vi "nanocal -- nuclear schottky fit V8.vi"() -> ()   [LabVIEW 2021] (continued)
\"mm1\" -> 0.000097559485   ,  \"mm2\" -> 0.023589285914   ,  \"mm3\" -> 0.055607523989   ,  \"T\" -> 0.360000000000   ,  \"B\" -> 8.000000000000   ,  \"θ\" -> 0.000000000000   ,  \"Reoff\" -> -3448979.591836734680   ,  \"Imoff\" -> 0.000000000000   ,  \"στ1\" -> 0.000376669141   ,  \"στS\" -> 0.000017301947   ,  \"στN\" -> 0.000201176295   ,  \"τ11 \" -> 0.000000000000   ,  \"τ12\" -> 0.000000000000   ,  \"τ22\" -> 0.000000000000   ,  \"τN1\" -> 0.000000000000   ,  \"τN2\" -> 0.000000000000   ,  \"σηlogτ1 \" -> 0.000000000000   ,  \"σηlogτS\" -> 0.000000000000   ,  \"σηlogτN\" -> 0.000000000000   ,  \"σlogτ1\" -> 0.000000000000   ,  \"σlogτS\" -> 0.000000000000   ,  \"σlogτN\" -> 0.000000000000   ,  \"σητ1\" -> 0.000000000000   ,  \"σητS \" -> 0.000000000000   ,  \"σητN\" -> 0.000000000000    |>   , \r\"IDS0383_210910_RAW_cal__sam_\" ->   <|    \"ζ\" -> 0.038341835326   ,  \"τ1\" -> 0.050866858713   ,  \"τS\" -> 0.030652081909   ,  \"τN\" -> 0.004623805952   ,  \"τC\" -> 0.002823684758   ,  \"κ0\" -> 0.000000002289   ,  \"mm1\" -> 0.000096034779   ,  \"mm2\" -> 0.028459102290   ,  \"mm3\" -> 0.061763836547   ,  \"T\" -> 0.360000000000   ,  \"B\" -> 8.000000000000   ,  \"θ\" -> 0.000000000000   ,  \"Reoff\" -> 0.000000000000   ,  \"Imoff\" -> 0.000000000000   ,  \"στ1\" -> 0.000000000000   ,  \"στS\" -> 0.000000000000   ,  \"στN\" -> 0.000000000000   ,  \"τ11 \" -> 0.000000000000   ,  \"τ12\" -> 0.000000000000   ,  \"τ22\" -> 0.000000000000   ,  \"τN1\" -> 0.000000000000   ,  \"τN2\" -> 0.000000000000   ,  \"σηlogτ1 \" -> 0.000000000000   ,  \"σηlogτS\" -> 0.000000000000   ,  \"σηlogτN\" -> 0.000000000000   ,  \"σlogτ1\" -> 0.000000000000   ,  \"σlogτS\" -> 0.000000000000   ,  \"σlogτN\" -> 0.000000000000   ,  \"σητ1\" -> 0.000000000000   ,  \"σητS \" -> 0.000000000000   ,  \"σητN\" -> 0.000000000000    |>   , \r\"IDS0384_210910_RAW_cal__ref_\" ->   <|    \"ζ\" -> 0.048414028377   ,  \"τ1\" -> 0.045010611313   ,  \"τS\" -> 0.024057574241   ,  \"τN\" -> 0.002275401127   ,  \"τC\" -> 0.001753445489   ,  \"κ0\" -> 0.000000002628   ,  \"mm1\" -> 0.000075920940   ,  \"mm2\" -> 0.024140914114   ,  \"mm3\" -> 0.050155082533   ,  \"T\" -> 0.430000000000   ,  \"B\" -> 8.000000000000   ,  \"θ\" -> 0.000000000000   ,  \"Reoff\" -> -3244897.959183673380   ,  \"Imoff\" -> 0.000000000000   ,  \"στ1\" -> 0.000665063032   ,  \"στS\" -> 0.000021368158   ,  \"στN\" -> 0.000342578343   ,  \"τ11 \" -> 0.000000000000   ,  \"τ12\" -> 0.000000000000   ,  \"τ22\" -> 0.000000000000   ,  \"τN1\" -> 0.000000000000   ,  \"τN2\" -> 0.000000000000   ,  \"σηlogτ1 \" -> 0.000000000000   ,  \"σηlogτS\" -> 0.000000000000   ,  \"σηlogτN\" -> 0.000000000000   ,  \"σlogτ1\" -> 0.000000000000   ,  \"σlogτS\" -> 0.000000000000   ,  \"σlogτN\" -> 0.000000000000   ,  \"σητ1\" -> 0.000000000000   ,  \"σητS \" -> 0.000000000000   ,  \"σητN\" -> 0.000000000000    |>   , \r\"IDS0384_210910_RAW_cal__sam_\" ->   <|    \"ζ\" -> 0.029950572027   ,  \"τ1\" -> 0.044923259835   ,  \"τS\" -> 0.030416367718   ,  \"τN\" -> 0.002541256331   ,  \"τC\" -> 0.003331031560   ,  \"κ0\" -> 0.000000002858   ,  \"mm1\" -> 0.000087776347   ,  \"mm2\" -> 0.029544080465   ,  \"mm3\" -> 0.052567158325   ,  \"T\" -> 0.430000000000   ,  \"B\" -> 8.000000000000   ,  \"θ\" -> 0.000000000000   ,  \"Reoff\" -> 0.000000000000   ,  \"Imoff\" -> 0.000000000000   ,  \"στ1\" -> 0.000000000000   ,  \"στS\" -> 0.000000000000   ,  \"στN\" -> 0.000000000000   ,  \"τ11 \" -> 0.000000000000   ,  \"τ12\" -> 0.000000000000   ,  \"τ22\" -> 0.000000000000   ,  \"τN1\" -> 0.000000000000   ,  \"τN2\" -> 0.000000000000   ,  \"σηlogτ1 \" -> 0.000000000000   ,  \"σηlogτS\" -> 0.000000000000   ,  \"σηlogτN\" -> 0.000000000000   ,  \"σlogτ1\" -> 0.000000000000   ,  \"σlogτS\" -> 0.000000000000   ,  \"σlogτN\" -> 0.000000000000   ,  \"σητ1\" -> 0.000000000000   ,  \"σητS \" -> 0.000000000000   ,  \"σητN\" -> 0.000000000000    |>   , \r\"IDS0385_210910_RAW_cal__ref_\" ->   <|    \"ζ\" -> 0.037803233744   ,  \"τ1\" -> 0.038048590559   ,  \"τS\" -> 0.025073667725   ,  \"τN\" -> 0.001214857209   ,  \"τC\" -> 0.002021423784   ,  \"κ0\" -> 0.000000003274   ,  \"mm1\" -> 0.000068491984   ,  \"mm2\" -> 0.025433188254   ,  \"mm3\" -> 0.041850650292   ,  \"T\" -> 0.530000000000   ,  \"B\" -> 8.000000000000   ,  \"θ\" -> 0.000000000000   ,  \"Reoff\" -> -1979591.836734693500   ,  \"Imoff\" -> 0.000000000000   ,  \"στ1\" -> 0.001496353936   ,  \"στS\" -> 0.000028774209   ,  \"στN\" -> 0.000698641170   ,  \"τ11 \" -> 0.000000000000   ,  \"τ12\" -> 0.000000000000   ,  \"τ22\" -> 0.000000000000   ,  \"τN1\" -> 0.000000000000   ,  \"τN2\" -> 0.000000000000   ,  \"σηlogτ1 \" -> 0.000000000000   ,  \"σηlogτS\" -> 0.000000000000   ,  \"σηlogτN\" -> 0.000000000000   ,  \"σlogτ1\" -> 0.000000000000   ,  \"σlogτS\" -> 0.000000000000   ,  \"σlogτN\" -> 0.000000000000   ,  \"σητ1\" -> 0.000000000000   ,  \"σητS \" -> 0.000000000000   ,  \"σητN\" -> 0.000000000000    |>   , \r\"IDS0385_210910_RAW_cal__sam_\" ->   <|    \"ζ\" -> 0.024600756648   ,  \"τ1\" -> 0.043958236582   ,  \"τS\" -> 0.031312750224   ,  \"τN\" -> 0.001348105931   ,  \"τC\" -> 0.003635120795   ,  \"κ0\" -> 0.000000003548   ,  \"mm1\" -> 0.000078569164   ,  \"mm2\" -> 0.031960914170   ,  \"mm3\" -> 0.049018211972   ,  \"T\" -> 0.530000000000   ,  \"B\" -> 8.000000000000   ,  \"θ\" -> 0.000000000000   ,  \"Reoff\" -> 0.000000000000   ,  \"Imoff\" -> 0.000000000000   ,  \"στ1\" -> 0.000000000000   ,  \"στS\" -> 0.000000000000   ,  \"στN\" -> 0.000000000000   ,  \"τ11 \" -> 0.000000000000   ,  \"τ12\" -> 0.000000000000   ,  \"τ22\" -> 0.000000000000   ,  \"τN1\" -> 0.000000000000   ,  \"τN2\" -> 0.000000000000   ,  \"σηlogτ1 \" -> 0.000000000000   ,  \"σηlogτS\" -> 0.000000000000   ,  \"σηlogτN\" -> 0.000000000000   ,  \"σlogτ1\" -> 0.000000000000   ,  \"σlogτS\" -> 0.000000000000   ,  \"σlogτN\" -> 0.000000000000   ,  \"σητ1\" -> 0.000000000000   ,  \"σητS \" -> 0.000000000000   ,  \"σητN\" -> 0.000000000000    |>   , \r\"IDS0386_210910_RAW_cal__ref_\" ->   <|    \"ζ\" -> 0.027746649612   ,  \"τ1\" -> 0.033747008640   ,  \"τS\" -> 0.026895844648   ,  \"τN\" -> 0.000802809162   ,  \"τC\" -> 0.002381968002   ,  \"κ0\" -> 0.000000003893   ,  \"mm1\" -> 0.000059322452   ,  \"mm2\" -> 0.026788808143   ,  \"mm3\" -> 0.037748044699   ,  \"T\" -> 0.630000000000   ,  \"B\" -> 8.000000000000   ,  \"θ\" -> 0.000000000000   ,  \"Reoff\" -> -918367.346938774919   ,  \"Imoff\" -> 0.000000000000   ,  \"στ1\" -> 0.002776813512   ,  \"στS\" -> 0.000037245612   ,  \"στN\" -> 0.001225903353   ,  \"τ11 \" -> 0.000000000000   ,  \"τ12\" -> 0.000000000000   ,  \"τ22\" -> 0.000000000000   ,  \"τN1\" -> 0.000000000000   ,  \"τN2\" -> 0.000000000000   ,  \"σηlogτ1 \" -> 0.000000000000   ,  \"σηlogτS\" -> 0.000000000000   ,  \"σηlogτN\" -> 0.000000000000   ,  \"σlogτ1\" -> 0.000000000000   ,  \"σlogτS\" -> 0.000000000000   ,  \"σlogτN\" -> 0.000000000000   ,  \"σητ1\" -> 0.000000000000   ,  \"σητS \" -> 0.000000000000   ,  \"σητN\" -> 0.000000000000    |>   , \r\"IDS0386_210910_RAW_cal__sam_\" ->   <|    \"ζ\" -> 0.019494767421   ,  \"τ1\" -> 0.040349410363   ,  \"τS\" -> 0.033202805363   ,  \"τN\" -> 0.000770756985   ,  \"τC\" -> 0.004303152006   ,  \"κ0\" -> 0.000000004241   ,  \"mm1\" -> 0.000073144130   ,  \"mm2\" -> 0.033928832906   ,  \"mm3\" -> 0.045286454378   ,  \"T\" -> 0.630000000000   ,  \"B\" -> 8.000000000000   ,  \"θ\" -> 0.000000000000   ,  \"Reoff\" -> 0.000000000000   ,  \"Imoff\" -> 0.000000000000   ,  \"στ1\" -> 0.000000000000   ,  \"στS\" -> 0.000000000000   ,  \"στN\" -> 0.000000000000   ,  \"τ11 \" -> 0.000000000000   ,  \"τ12\" -> 0.000000000000   ,  \"τ22\" -> 0.000000000000   ,  \"τN1\" -> 0.000000000000   ,  \"τN2\" -> 0.000000000000   ,  \"σηlogτ1 \" -> 0.000000000000   ,  \"σηlogτS\" -> 0.000000000000   ,  \"σηlogτN\" -> 0.000000000000   ,  \"σlogτ1\" -> 0.000000000000   ,  \"σlogτS\" -> 0.000000000000   ,  \"σlogτN\" -> 0.000000000000   ,  \"σητ1\" -> 0.000000000000   ,  \"σητS \" -> 0.000000000000   ,  \"σητN\" -> 0.000000000000    |>   , \r\"IDS0387_210910_RAW_cal__ref_\" ->   <|    \"ζ\" -> 0.019313601846   ,  \"τ1\" -> 0.030127940029   ,  \"τS\" -> 0.030834079671   ,  \"τN\" -> 0.000314036282   ,  \"τC\" -> 0.003752610189   ,  \"κ0\" -> 0.000000005418   ,  \"mm1\" -> 0.000063634095   ,  \"mm2\" -> 0.028697652257   ,  \"mm3\" -> 0.036868962129   ,  \"T\" -> 0.830000000000   ,  \"B\" -> 8.000000000000   ,  \"θ\" -> 0.000000000000   ,  \"Reoff\" -> -265306.122448978945   ,  \"Imoff\" -> 0.000000000000   ,  \"στ1\" -> 0.011424377975   ,  \"στS\" -> 0.000061541841   ,  \"στN\" -> 0.005052534408   ,  \"τ11 \" -> 0.000000000000   ,  \"τ12\" -> 0.000000000000   ,  \"τ22\" -> 0.000000000000   ,  \"τN1\" -> 0.000000000000   ,  \"τN2\" -> 0.000000000000   ,  \"σηlogτ1 \" -> 0.000000000000   ,  \"σηlogτS\" -> 0.000000000000   ,  \"σηlogτN\" -> 0.000000000000   ,  \"σlogτ1\" -> 0.000000000000   ,  \"σlogτS\" -> 0.000000000000   ,  \"σlogτN\" -> 0.000000000000   ,  \"σητ1\" -> 0.000000000000   ,  \"σητS \" -> 0.000000000000   ,  \"σητN\" -> 0.000000000000    |>   , \r\"IDS0387_210910_RAW_cal__sam_\" ->   <|    \"ζ\" -> 0.013958531253   ,  \"τ1\" -> 0.040449551738   ,  \"τS\" -> 0.038075316972   ,  \"τN\" -> 0.000218997482   ,  \"τC\" -> 0.005348147372   ,  \"κ0\" -> 0.000000005866   ,  \"mm1\" -> 0.000064761782   ,  \"mm2\" -> 0.038768935960   ,  \"mm3\" -> 0.045792848207   ,  \"T\" -> 0.830000000000   ,  \"B\" -> 8.000000000000   ,  \"θ\" -> 0.000000000000   ,  \"Reoff\" -> 0.000000000000   ,  \"Imoff\" -> 0.000000000000   ,  \"στ1\" -> 0.000000000000   ,  \"στS\" -> 0.000000000000   ,  \"στN\" -> 0.000000000000   ,  \"τ11 \" -> 0.000000000000   ,  \"τ12\" -> 0.000000000000   ,  \"τ22\" -> 0.000000000000   ,  \"τN1\" -> 0.000000000000   ,  \"τN2\" -> 0.000000000000   ,  \"σηlogτ1 \" -> 0.000000000000   ,  \"σηlogτS\" -> 0.000000000000   ,  \"σηlogτN\" -> 0.000000000000   ,  \"σlogτ1\" -> 0.000000000000   ,  \"σlogτS\" -> 0.000000000000   ,  \"σlogτN\" -> 0.000000000000   ,  \"σητ1\" -> 0.000000000000   ,  \"σητS \" -> 0.000000000000   ,  \"σητN\" -> 0.000000000000    |>   , \r\"IDS0388_210910_RAW_cal__ref_\" ->   <|    \"ζ\" -> 0.016319215592   ,  \"τ1\" -> 0.028476907475   ,  \"τS\" -> 0.040634863110   ,  \"τN\" -> 0.000119778793   ,  \"τC\" -> 0.003363489331   ,  \"κ0\" -> 0.000000007540   ,  \"mm1\" -> 0.000049996694   ,  \"mm2\" -> 0.028266417043   ,  \"mm3\" -> 0.044943708759   ,  \"T\" -> 1.130000000000   ,  \"B\" -> 8.000000000000   ,  \"θ\" -> 0.000000000000   ,  \"Reoff\" -> -428571.428571428172   ,  \"Imoff\" -> 0.000000000000   ,  \"στ1\" -> 0.056097814520   ,  \"στS\" -> 0.000101338732   ,  \"στN\" -> 0.027741009439   ,  \"τ11 \" -> 0.000000000000   ,  \"τ12\" -> 0.000000000000   ,  \"τ22\" -> 0.000000000000   ,  \"τN1\" -> 0.000000000000   ,  \"τN2\" -> 0.000000000000   ,  \"σηlogτ1 \" -> 0.000000000000   ,  \"σηlogτS\" -> 0.000000000000   ,  \"σηlogτN\" -> 0.000000000000   ,  \"σlogτ1\" -> 0.000000000000   ,  \"σlogτS\" -> 0.000000000000   ,  \"σlogτN\" -> 0.000000000000   ,  \"σητ1\" -> 0.000000000000   ,  \"σητS \" -> 0.000000000000   ,  \"σητN\" -> 0.000000000000    |>   , \r\"IDS0388_210910_RAW_cal__sam_\" ->   <|    \"ζ\" -> 0.011551866824   ,  \"τ1\" -> 0.040411227639   ,  \"τS\" -> 0.048181354691   ,  \"τN\" -> 0.000103559724   ,  \"τC\" -> 0.006232382617   ,  \"κ0\" -> 0.000000008161   ,  \"mm1\" -> 0.000063176601   ,  \"mm2\" -> 0.040126882627   ,  \"mm3\" -> 0.055296246344   ,  \"T\" -> 1.130000000000   ,  \"B\" -> 8.000000000000   ,  \"θ\" -> 0.000000000000   ,  \"Reoff\" -> 0.000000000000   ,  \"Imoff\" -> 0.000000000000   ,  \"στ1\" -> 0.000000000000   ,  \"στS\" -> 0.000000000000   ,  \"στN\" -> 0.000000000000   ,  \"τ11 \" -> 0.000000000000   ,  \"τ12\" -> 0.000000000000   ,  \"τ22\" -> 0.000000000000   ,  \"τN1\" -> 0.000000000000   ,  \"τN2\" -> 0.000000000000   ,  \"σηlogτ1 \" -> 0.000000000000   ,  \"σηlogτS\" -> 0.000000000000   ,  \"σηlogτN\" -> 0.000000000000   ,  \"σlogτ1\" -> 0.000000000000   ,  \"σlogτS\" -> 0.000000000000   ,  \"σlogτN\" -> 0.000000000000   ,  \"σητ1\" -> 0.000000000000   ,  \"σητS \" -> 0.000000000000   ,  \"σητN\" -> 0.000000000000    |>   , \r\"IDS0389_210910_RAW_cal__ref_\" ->   <|    \"ζ\" -> 0.019598304636   ,  \"τ1\" -> 0.026919422871   ,  \"τS\" -> 0.016301457757   ,  \"τN\" -> 0.000045685674   ,  \"τC\" -> 0.003967911941   ,  \"κ0\" -> 0.000000010417   ,  \"mm1\" -> 0.000061755971   ,  \"mm2\" -> 0.020381971483   ,  \"mm3\" -> 0.027111127086   ,  \"T\" -> 1.520000000000   ,  \"B\" -> 8.000000000000   ,  \"θ\" -> 0.000000000000   ,  \"Reoff\" -> -551020.408163265324   ,  \"Imoff\" -> 0.000000000000   ,  \"στ1\" -> 0.092677427953   ,  \"στS\" -> 0.000105745650   ,  \"στN\" -> 0.043266676347   ,  \"τ11 \" -> 0.000000000000   ,  \"τ12\" -> 0.000000000000   ,  \"τ22\" -> 0.000000000000   ,  \"τN1\" -> 0.000000000000   ,  \"τN2\" -> 0.000000000000   ,  \"σηlogτ1 \" -> 0.000000000000   ,  \"σηlogτS\" -> 0.000000000000   ,  \"σηlogτN\" -> 0.000000000000   ,  \"σlogτ1\" -> 0.000000000000   ,  \"σlogτS\" -> 0.000000000000   ,  \"σlogτN\" -> 0.000000000000   ,  \"σητ1\" -> 0.000000000000   ,  \"σητS \" -> 0.000000000000   ,  \"σητN\" -> 0.000000000000    |>   , \r\"IDS0389_210910_RAW_cal__sam_\" ->   <|    \"ζ\" -> 0.011148198813   ,  \"τ1\" -> 0.038849151842   ,  \"τS\" -> 0.019213865355   ,  \"τN\" -> 0.000045035153   ,  \"τC\" -> 0.005536708133   ,  \"κ0\" -> 0.000000011229   ,  \"mm1\" -> 0.000047596165   ,  \"mm2\" -> 0.024836509281   ,  \"mm3\" -> 0.038975357089   ,  \"T\" -> 1.520000000000   ,  \"B\" -> 8.000000000000   ,  \"θ\" -> 0.000000000000   ,  \"Reoff\" -> 0.000000000000   ,  \"Imoff\" -> 0.000000000000   ,  \"στ1\" -> 0.000000000000   ,  \"στS\" -> 0.000000000000   ,  \"στN\" -> 0.000000000000   ,  \"τ11 \" -> 0.000000000000   ,  \"τ12\" -> 0.000000000000   ,  \"τ22\" -> 0.000000000000   ,  \"τN1\" -> 0.000000000000   ,  \"τN2\" -> 0.000000000000   ,  \"σηlogτ1 \" -> 0.000000000000   ,  \"σηlogτS\" -> 0.000000000000   ,  \"σηlogτN\" -> 0.000000000000   ,  \"σlogτ1\" -> 0.000000000000   ,  \"σlogτS\" -> 0.000000000000   ,  \"σlogτN\" -> 0.000000000000   ,  \"σητ1\" -> 0.000000000000   ,  \"σητS \" -> 0.000000000000   ,  \"σητN\" -> 0.000000000000    |>   , \r\"IDS0390_210910_RAW_cal__ref_\" ->   <|    \"ζ\" -> 0.016930911493   ,  \"τ1\" -> 0.024035041541   ,  \"τS\" -> 0.011182752166   ,  \"τN\" -> 0.000024854278   ,  \"τC\" -> 0.003445627696   ,  \"κ0\" -> 0.000000013051   ,  \"mm1\" -> 0.000044158259   ,  \"mm2\" -> 0.014733556006   ,  \"mm3\" -> 0.024100316408   ,  \"T\" -> 1.900000000000   ,  \"B\" -> 8.000000000000   ,  \"θ\" -> 0.000000000000   ,  \"Reoff\" -> -346938.775510204024   ,  \"Imoff\" -> 0.000000000000   ,  \"στ1\" -> 0.156695414704   ,  \"στS\" -> 0.000120966838   ,  \"στN\" -> 0.078791038522   ,  \"τ11 \" -> 0.000000000000   ,  \"τ12\" -> 0.000000000000   ,  \"τ22\" -> 0.000000000000   ,  \"τN1\" -> 0.000000000000   ,  \"τN2\" -> 0.000000000000   ,  \"σηlogτ1 \" -> 0.000000000000   ,  \"σηlogτS\" -> 0.000000000000   ,  \"σηlogτN\" -> 0.000000000000   ,  \"σlogτ1\" -> 0.000000000000   ,  \"σlogτS\" -> 0.000000000000   ,  \"σlogτN\" -> 0.000000000000   ,  \"σητ1\" -> 0.000000000000   ,  \"σητS \" -> 0.000000000000   ,  \"σητN\" -> 0.000000000000    |>   , \r\"IDS0390_210910_RAW_cal__sam_\" ->   <|    \"ζ\" -> 0.010826949430   ,  \"τ1\" -> 0.038768037521   ,  \"τS\" -> 0.012925317198   ,  \"τN\" -> 0.000029157336   ,  \"τC\" -> 0.005196063884   ,  \"κ0\" -> 0.000000013864   ,  \"mm1\" -> 0.000039906108   ,  \"mm2\" -> 0.018195372076   ,  \"mm3\" -> 0.038823555195   ,  \"T\" -> 1.900000000000   ,  \"B\" -> 8.000000000000   ,  \"θ\" -> 0.000000000000   ,  \"Reoff\" -> 0.000000000000   ,  \"Imoff\" -> 0.000000000000   ,  \"στ1\" -> 0.000000000000   ,  \"στS\" -> 0.000000000000   ,  \"στN\" -> 0.000000000000   ,  \"τ11 \" -> 0.000000000000   ,  \"τ12\" -> 0.000000000000   ,  \"τ22\" -> 0.000000000000   ,  \"τN1\" -> 0.000000000000   ,  \"τN2\" -> 0.000000000000   ,  \"σηlogτ1 \" -> 0.000000000000   ,  \"σηlogτS\" -> 0.000000000000   ,  \"σηlogτN\" -> 0.000000000000   ,  \"σlogτ1\" -> 0.000000000000   ,  \"σlogτS\" -> 0.000000000000   ,  \"σlogτN\" -> 0.000000000000   ,  \"σητ1\" -> 0.000000000000   ,  \"σητS \" -> 0.000000000000   ,  \"σητN\" -> 0.000000000000    |>   , \r\"IDS0391_210910_RAW_cal__ref_\" ->   <|    \"ζ\" -> 0.014199379988   ,  \"τ1\" -> 0.031876047451   ,  \"τS\" -> 0.042500159356   ,  \"τN\" -> 0.000092944151   ,  \"τC\" -> 0.003599424306   ,  \"κ0\" -> 0.000000008340   ,  \"mm1\" -> 0.000046556540   ,  \"mm2\" -> 0.031676737878   ,  \"mm3\" -> 0.046950076508   ,  \"T\" -> 1.250000000000   ,  \"B\" -> 8.000000000000   ,  \"θ\" -> 0.000000000000   ,  \"Reoff\" -> -224489.795918366871   ,  \"Imoff\" -> 0.000000000000   ,  \"στ1\" -> 0.081986423861   ,  \"στS\" -> 0.000106847397   ,  \"στN\" -> 0.039114279615   ,  \"τ11 \" -> 0.000000000000   ,  \"τ12\" -> 0.000000000000   ,  \"τ22\" -> 0.000000000000   ,  \"τN1\" -> 0.000000000000   ,  \"τN2\" -> 0.000000000000   ,  \"σηlogτ1 \" -> 0.000000000000   ,  \"σηlogτS\" -> 0.000000000000   ,  \"σηlogτN\" -> 0.000000000000   ,  \"σlogτ1\" -> 0.000000000000   ,  \"σlogτS\" -> 0.000000000000   ,  \"σlogτN\" -> 0.000000000000   ,  \"σητ1\" -> 0.000000000000   ,  \"σητS \" -> 0.000000000000   ,  \"σητN\" -> 0.000000000000    |>   , \r\"IDS0391_210910_RAW_cal__sam_\" ->   <|    \"ζ\" -> 0.010962610928   ,  \"τ1\" -> 0.040398807374   ,  \"τS\" -> 0.051328988590   ,  \"τN\" -> 0.000070281011   ,  \"τC\" -> 0.006422533164   ,  \"κ0\" -> 0.000000008958   ,  \"mm1\" -> 0.000062039854   ,  \"mm2\" -> 0.040240103995   ,  \"mm3\" -> 0.058481936484   ,  \"T\" -> 1.250000000000   ,  \"B\" -> 8.000000000000   ,  \"θ\" -> 0.000000000000   ,  \"Reoff\" -> 0.000000000000   ,  \"Imoff\" -> 0.000000000000   ,  \"στ1\" -> 0.000000000000   ,  \"στS\" -> 0.000000000000   ,  \"στN\" -> 0.000000000000   ,  \"τ11 \" -> 0.000000000000   ,  \"τ12\" -> 0.000000000000   ,  \"τ22\" -> 0.000000000000   ,  \"τN1\" -> 0.000000000000   ,  \"τN2\" -> 0.000000000000   ,  \"σηlogτ1 \" -> 0.000000000000   ,  \"σηlogτS\" -> 0.000000000000   ,  \"σηlogτN\" -> 0.000000000000   ,  \"σlogτ1\" -> 0.000000000000   ,  \"σlogτS\" -> 0.000000000000   ,  \"σlogτN\" -> 0.000000000000   ,  \"σητ1\" -> 0.000000000000   ,  \"σητS \" -> 0.000000000000   ,  \"σητN\" -> 0.000000000000    |>   , \r\"IDS0392_210910_RAW_cal__ref_\" ->   <|    \"ζ\" -> 0.015881193155   ,  \"τ1\" -> 0.030137709791   ,  \"τS\" -> 0.030744706039   ,  \"τN\" -> 0.000065162997   ,  \"τC\" -> 0.003875572630   ,  \"κ0\" -> 0.000000009446   ,  \"mm1\" -> 0.000053981464   ,  \"mm2\" -> 0.029765266989   ,  \"mm3\" -> 0.035493200486   ,  \"T\" -> 1.390000000000   ,  \"B\" -> 8.000000000000   ,  \"θ\" -> 0.000000000000   ,  \"Reoff\" -> -224489.795918366871   ,  \"Imoff\" -> 0.000000000000   ,  \"στ1\" -> 0.096426784918   ,  \"στS\" -> 0.000107023117   ,  \"στN\" -> 0.042599463915   ,  \"τ11 \" -> 0.000000000000   ,  \"τ12\" -> 0.000000000000   ,  \"τ22\" -> 0.000000000000   ,  \"τN1\" -> 0.000000000000   ,  \"τN2\" -> 0.000000000000   ,  \"σηlogτ1 \" -> 0.000000000000   ,  \"σηlogτS\" -> 0.000000000000   ,  \"σηlogτN\" -> 0.000000000000   ,  \"σlogτ1\" -> 0.000000000000   ,  \"σlogτS\" -> 0.000000000000   ,  \"σlogτN\" -> 0.000000000000   ,  \"σητ1\" -> 0.000000000000   ,  \"σητS \" -> 0.000000000000   ,  \"σητN\" -> 0.000000000000    |>   , \r\"IDS0392_210910_RAW_cal__sam_\" ->   <|    \"ζ\" -> 0.010962610928   ,  \"τ1\" -> 0.040398807374   ,  \"τS\" -> 0.051328988590   ,  \"τN\" -> 0.000070281011   ,  \"τC\" -> 0.006422533164   ,  \"κ0\" -> 0.000000008958   ,  \"mm1\" -> 0.000062039854   ,  \"mm2\" -> 0.040240103995   ,  \"mm3\" -> 0.058481936484   ,  \"T\" -> 1.390000000000   ,  \"B\" -> 8.000000000000   ,  \"θ\" -> 0.000000000000   ,  \"Reoff\" -> 0.000000000000   ,  \"Imoff\" -> 0.000000000000   ,  \"στ1\" -> 0.000000000000   ,  \"στS\" -> 0.000000000000   ,  \"στN\" -> 0.000000000000   ,  \"τ11 \" -> 0.000000000000   ,  \"τ12\" -> 0.000000000000   ,  \"τ22\" -> 0.000000000000   ,  \"τN1\" -> 0.000000000000   ,  \"τN2\" -> 0.000000000000   ,  \"σηlogτ1 \" -> 0.000000000000   ,  \"σηlogτS\" -> 0.000000000000   ,  \"σηlogτN\" -> 0.000000000000   ,  \"σlogτ1\" -> 0.000000000000   ,  \"σlogτS\" -> 0.000000000000   ,  \"σlogτN\" -> 0.000000000000   ,  \"σητ1\" -> 0.000000000000   ,  \"σητS \" -> 0.000000000000   ,  \"σητN\" -> 0.000000000000    |>   , \r\"IDS0393_210910_RAW_cal__ref_\" ->   <|    \"ζ\" -> 0.015265277738   ,  \"τ1\" -> 0.021483559008   ,  \"τS\" -> 0.008480397220   ,  \"τN\" -> 0.000005157300   ,  \"τC\" -> 0.002746236022   ,  \"κ0\" -> 0.000000023389   ,  \"mm1\" -> 0.000031392950   ,  \"mm2\" -> 0.011318870449   ,  \"mm3\" -> 0.021494620498   ,  \"T\" -> 3.110000000000   ,  \"B\" -> 8.000000000000   ,  \"θ\" -> 0.000000000000   ,  \"Reoff\" -> -183673.469387754798   ,  \"Imoff\" -> 0.000000000000   ,  \"στ1\" -> 1.099539205985   ,  \"στS\" -> 0.000204841984   ,  \"στN\" -> 0.599548494837   ,  \"τ11 \" -> 0.000000000000   ,  \"τ12\" -> 0.000000000000   ,  \"τ22\" -> 0.000000000000   ,  \"τN1\" -> 0.000000000000   ,  \"τN2\" -> 0.000000000000   ,  \"σηlogτ1 \" -> 0.000000000000   ,  \"σηlogτS\" -> 0.000000000000   ,  \"σηlogτN\" -> 0.000000000000   ,  \"σlogτ1\" -> 0.000000000000   ,  \"σlogτS\" -> 0.000000000000   ,  \"σlogτN\" -> 0.000000000000   ,  \"σητ1\" -> 0.000000000000   ,  \"σητS \" -> 0.000000000000   ,  \"σητN\" -> 0.000000000000    |>   , \r\"IDS0393_210910_RAW_cal__sam_\" ->   <|    \"ζ\" -> 0.010962610928   ,  \"τ1\" -> 0.040398807374   ,  \"τS\" -> 0.051328988590   ,  \"τN\" -> 0.000070281011   ,  \"τC\" -> 0.006422533164   ,  \"κ0\" -> 0.000000008958   ,  \"mm1\" -> 0.000062039854   ,  \"mm2\" -> 0.040240103995   ,  \"mm3\" -> 0.058481936484   ,  \"T\" -> 3.110000000000   ,  \"B\" -> 8.000000000000   ,  \"θ\" -> 0.000000000000   ,  \"Reoff\" -> 0.000000000000   ,  \"Imoff\" -> 0.000000000000   ,  \"στ1\" -> 0.000000000000   ,  \"στS\" -> 0.000000000000   ,  \"στN\" -> 0.000000000000   ,  \"τ11 \" -> 0.000000000000   ,  \"τ12\" -> 0.000000000000   ,  \"τ22\" -> 0.000000000000   ,  \"τN1\" -> 0.000000000000   ,  \"τN2\" -> 0.000000000000   ,  \"σηlogτ1 \" -> 0.000000000000   ,  \"σηlogτS\" -> 0.000000000000   ,  \"σηlogτN\" -> 0.000000000000   ,  \"σlogτ1\" -> 0.000000000000   ,  \"σlogτS\" -> 0.000000000000   ,  \"σlogτN\" -> 0.000000000000   ,  \"σητ1\" -> 0.000000000000   ,  \"σητS \" -> 0.000000000000   ,  \"σητN\" -> 0.000000000000    |>   , \r\"IDS0394_210910_RAW_cal__ref_\" ->   <|    \"ζ\" -> 0.016150664037   ,  \"τ1\" -> 0.020476039479   ,  \"τS\" -> 0.005934845736   ,  \"τN\" -> 0.000000659524   ,  \"τC\" -> 0.001816691327   ,  \"κ0\" -> 0.000000058090   ,  \"mm1\" -> 0.000022253026   ,  \"mm2\" -> 0.007824721591   ,  \"mm3\" -> 0.020477123801   ,  \"T\" -> 5.750000000000   ,  \"B\" -> 8.000000000000   ,  \"θ\" -> 0.000000000000   ,  \"Reoff\" -> -61224.489795917645   ,  \"Imoff\" -> 0.000000000000   ,  \"στ1\" -> 17.464261644387   ,  \"στS\" -> 0.000446907236   ,  \"στN\" -> 11.183810891776   ,  \"τ11 \" -> 0.000000000000   ,  \"τ12\" -> 0.000000000000   ,  \"τ22\" -> 0.000000000000   ,  \"τN1\" -> 0.000000000000   ,  \"τN2\" -> 0.000000000000   ,  \"σηlogτ1 \" -> 0.000000000000   ,  \"σηlogτS\" -> 0.000000000000   ,  \"σηlogτN\" -> 0.000000000000   ,  \"σlogτ1\" -> 0.000000000000   ,  \"σlogτS\" -> 0.000000000000   ,  \"σlogτN\" -> 0.000000000000   ,  \"σητ1\" -> 0.000000000000   ,  \"σητS \" -> 0.000000000000   ,  \"σητN\" -> 0.000000000000    |>   , \r\"IDS0394_210910_RAW_cal__sam_\" ->   <|    \"ζ\" -> 0.010962610928   ,  \"τ1\" -> 0.040398807374   ,  \"τS\" -> 0.051328988590   ,  \"τN\" -> 0.000070281011   ,  \"τC\" -> 0.006422533164   ,  \"κ0\" -> 0.000000008958   ,  \"mm1\" -> 0.000062039854   ,  \"mm2\" -> 0.040240103995   ,  \"mm3\" -> 0.058481936484   ,  \"T\" -> 5.750000000000   ,  \"B\" -> 8.000000000000   ,  \"θ\" -> 0.000000000000   ,  \"Reoff\" -> 0.000000000000   ,  \"Imoff\" -> 0.000000000000   ,  \"στ1\" -> 0.000000000000   ,  \"στS\" -> 0.000000000000   ,  \"στN\" -> 0.000000000000   ,  \"τ11 \" -> 0.000000000000   ,  \"τ12\" -> 0.000000000000   ,  \"τ22\" -> 0.000000000000   ,  \"τN1\" -> 0.000000000000   ,  \"τN2\" -> 0.000000000000   ,  \"σηlogτ1 \" -> 0.000000000000   ,  \"σηlogτS\" -> 0.000000000000   ,  \"σηlogτN\" -> 0.000000000000   ,  \"σlogτ1\" -> 0.000000000000   ,  \"σlogτS\" -> 0.000000000000   ,  \"σlogτN\" -> 0.000000000000   ,  \"σητ1\" -> 0.000000000000   ,  \"σητS \" -> 0.000000000000   ,  \"σητN\" -> 0.000000000000    |>   , \r\"IDS0395_210910_RAW_cal__ref_\" ->   <|    \"ζ\" -> 0.014324372038   ,  \"τ1\" -> 0.026919249661   ,  \"τS\" -> 0.041101383750   ,  \"τN\" -> 0.000075874488   ,  \"τC\" -> 0.003639322080   ,  \"κ0\" -> 0.000000008618   ,  \"mm1\" -> 0.000047317902   ,  \"mm2\" -> 0.026807591507   ,  \"mm3\" -> 0.045470758936   ,  \"T\" -> 1.310000000000   ,  \"B\" -> 8.000000000000   ,  \"θ\" -> 0.000000000000   ,  \"Reoff\" -> -224489.795918366871   ,  \"Imoff\" -> 0.000000000000   ,  \"στ1\" -> 0.105285402428   ,  \"στS\" -> 0.000123348691   ,  \"στN\" -> 0.053591499241   ,  \"τ11 \" -> 0.000000000000   ,  \"τ12\" -> 0.000000000000   ,  \"τ22\" -> 0.000000000000   ,  \"τN1\" -> 0.000000000000   ,  \"τN2\" -> 0.000000000000   ,  \"σηlogτ1 \" -> 0.000000000000   ,  \"σηlogτS\" -> 0.000000000000   ,  \"σηlogτN\" -> 0.000000000000   ,  \"σlogτ1\" -> 0.000000000000   ,  \"σlogτS\" -> 0.000000000000   ,  \"σlogτN\" -> 0.000000000000   ,  \"σητ1\" -> 0.000000000000   ,  \"σητS \" -> 0.000000000000   ,  \"σητN\" -> 0.000000000000    |>   , \r\"IDS0395_210910_RAW_cal__sam_\" ->   <|    \"ζ\" -> 0.010962610928   ,  \"τ1\" -> 0.040398807374   ,  \"τS\" -> 0.051328988590   ,  \"τN\" -> 0.000070281011   ,  \"τC\" -> 0.006422533164   ,  \"κ0\" -> 0.000000008958   ,  \"mm1\" -> 0.000062039854   ,  \"mm2\" -> 0.040240103995   ,  \"mm3\" -> 0.058481936484   ,  \"T\" -> 1.310000000000   ,  \"B\" -> 8.000000000000   ,  \"θ\" -> 0.000000000000   ,  \"Reoff\" -> 0.000000000000   ,  \"Imoff\" -> 0.000000000000   ,  \"στ1\" -> 0.000000000000   ,  \"στS\" -> 0.000000000000   ,  \"στN\" -> 0.000000000000   ,  \"τ11 \" -> 0.000000000000   ,  \"τ12\" -> 0.000000000000   ,  \"τ22\" -> 0.000000000000   ,  \"τN1\" -> 0.000000000000   ,  \"τN2\" -> 0.000000000000   ,  \"σηlogτ1 \" -> 0.000000000000   ,  \"σηlogτS\" -> 0.000000000000   ,  \"σηlogτN\" -> 0.000000000000   ,  \"σlogτ1\" -> 0.000000000000   ,  \"σlogτS\" -> 0.000000000000   ,  \"σlogτN\" -> 0.000000000000   ,  \"σητ1\" -> 0.000000000000   ,  \"σητS \" -> 0.000000000000   ,  \"σητN\" -> 0.000000000000    |>   , \r\"IDS0407_220525_RAW_cal__ref_\" ->   <|    \"ζ\" -> 0.185082039484   ,  \"τ1\" -> 0.020077955798   ,  \"τS\" -> 0.012960000170   ,  \"τN\" -> 0.004537831890   ,  \"τC\" -> 0.001384950660   ,  \"κ0\" -> 0.000000000762   ,  \"mm1\" -> 0.000200762639   ,  \"mm2\" -> 0.010571518349   ,  \"mm3\" -> 0.031426991974   ,  \"T\" -> 0.200000000000   ,  \"B\" -> 0.000000000000   ,  \"θ\" -> 0.000000000000   ,  \"Reoff\" -> -36285714.285714283600   ,  \"Imoff\" -> 0.000000000000   ,  \"στ1\" -> 0.006379909660   ,  \"στS\" -> 0.001208627120   ,  \"στN\" -> 0.001505491002   ,  \"τ11 \" -> 0.000000000000   ,  \"τ12\" -> 0.000000000000   ,  \"τ22\" -> 0.000000000000   ,  \"τN1\" -> 0.000000000000   ,  \"τN2\" -> 0.000000000000   ,  \"σηlogτ1 \" -> 0.000000000000   ,  \"σηlogτS\" -> 0.000000000000   ,  \"σηlogτN\" -> 0.000000000000   ,  \"σlogτ1\" -> 0.000000000000   ,  \"σlogτS\" -> 0.000000000000   ,  \"σlogτN\" -> 0.000000000000   ,  \"σητ1\" -> 0.000000000000   ,  \"σητS \" -> 0.000000000000   ,  \"σητN\" -> 0.000000000000    |>   , \r\"IDS0407_220525_RAW_cal__sam_\" ->   <|    \"ζ\" -> 0.107728168967   ,  \"τ1\" -> 0.019656327090   ,  \"τS\" -> 0.016556579862   ,  \"τN\" -> 0.004758156992   ,  \"τC\" -> 0.001123654800   ,  \"κ0\" -> 0.000000000861   ,  \"mm1\" -> 0.000103510666   ,  \"mm2\" -> 0.011667063931   ,  \"mm3\" -> 0.032620341720   ,  \"T\" -> 0.200000000000   ,  \"B\" -> 0.000000000000   ,  \"θ\" -> 0.000000000000   ,  \"Reoff\" -> -36285714.285714283600   ,  \"Imoff\" -> 0.000000000000   ,  \"στ1\" -> 0.009912643228   ,  \"στS\" -> 0.001520300197   ,  \"στN\" -> 0.002063455636   ,  \"τ11 \" -> 0.000000000000   ,  \"τ12\" -> 0.000000000000   ,  \"τ22\" -> 0.000000000000   ,  \"τN1\" -> 0.000000000000   ,  \"τN2\" -> 0.000000000000   ,  \"σηlogτ1 \" -> 0.000000000000   ,  \"σηlogτS\" -> 0.000000000000   ,  \"σηlogτN\" -> 0.000000000000   ,  \"σlogτ1\" -> 0.000000000000   ,  \"σlogτS\" -> 0.000000000000   ,  \"σlogτN\" -> 0.000000000000   ,  \"σητ1\" -> 0.000000000000   ,  \"σητS \" -> 0.000000000000   ,  \"σητN\" -> 0.000000000000    |>   , \r\"IDS0408_220525_RAW_cal__ref_\" ->   <|    \"ζ\" -> 0.136667515629   ,  \"τ1\" -> 0.013397105369   ,  \"τS\" -> 0.011359937502   ,  \"τN\" -> 0.003646822051   ,  \"τC\" -> 0.000857952267   ,  \"κ0\" -> 0.000000001040   ,  \"mm1\" -> 0.000097405399   ,  \"mm2\" -> 0.007836148791   ,  \"mm3\" -> 0.023379199545   ,  \"T\" -> 0.250000000000   ,  \"B\" -> 0.000000000000   ,  \"θ\" -> 0.000000000000   ,  \"Reoff\" -> -36285714.285714283600   ,  \"Imoff\" -> 0.000000000000   ,  \"στ1\" -> 0.003212907599   ,  \"στS\" -> 0.000580541661   ,  \"στN\" -> 0.000811635824   ,  \"τ11 \" -> 0.000000000000   ,  \"τ12\" -> 0.000000000000   ,  \"τ22\" -> 0.000000000000   ,  \"τN1\" -> 0.000000000000   ,  \"τN2\" -> 0.000000000000   ,  \"σηlogτ1 \" -> 0.000000000000   ,  \"σηlogτS\" -> 0.000000000000   ,  \"σηlogτN\" -> 0.000000000000   ,  \"σlogτ1\" -> 0.000000000000   ,  \"σlogτS\" -> 0.000000000000   ,  \"σlogτN\" -> 0.000000000000   ,  \"σητ1\" -> 0.000000000000   ,  \"σητS \" -> 0.000000000000   ,  \"σητN\" -> 0.000000000000    |>   , \r\"IDS0408_220525_RAW_cal__sam_\" ->   <|    \"ζ\" -> 0.086238207773   ,  \"τ1\" -> 0.018354133297   ,  \"τS\" -> 0.015001679768   ,  \"τN\" -> 0.004138272742   ,  \"τC\" -> 0.001377972360   ,  \"κ0\" -> 0.000000001190   ,  \"mm1\" -> 0.000101440698   ,  \"mm2\" -> 0.010941566515   ,  \"mm3\" -> 0.029479646155   ,  \"T\" -> 0.250000000000   ,  \"B\" -> 0.000000000000   ,  \"θ\" -> 0.000000000000   ,  \"Reoff\" -> -26000000.000000000000   ,  \"Imoff\" -> 0.000000000000   ,  \"στ1\" -> 0.004778614510   ,  \"στS\" -> 0.000718856892   ,  \"στN\" -> 0.001132000122   ,  \"τ11 \" -> 0.000000000000   ,  \"τ12\" -> 0.000000000000   ,  \"τ22\" -> 0.000000000000   ,  \"τN1\" -> 0.000000000000   ,  \"τN2\" -> 0.000000000000   ,  \"σηlogτ1 \" -> 0.000000000000   ,  \"σηlogτS\" -> 0.000000000000   ,  \"σηlogτN\" -> 0.000000000000   ,  \"σlogτ1\" -> 0.000000000000   ,  \"σlogτS\" -> 0.000000000000   ,  \"σlogτN\" -> 0.000000000000   ,  \"σητ1\" -> 0.000000000000   ,  \"σητS \" -> 0.000000000000   ,  \"σητN\" -> 0.000000000000    |>   , \r\"IDS0409_220525_RAW_cal__ref_\" ->   <|    \"ζ\" -> 0.104307058542   ,  \"τ1\" -> 0.013891003970   ,  \"τS\" -> 0.010729497189   ,  \"τN\" -> 0.003200228441   ,  \"τC\" -> 0.001175856975   ,  \"κ0\" -> 0.000000001350   ,  \"mm1\" -> 0.000101815669   ,  \"mm2\" -> 0.008053188158   ,  \"mm3\" -> 0.022294551454   ,  \"T\" -> 0.300000000000   ,  \"B\" -> 0.000000000000   ,  \"θ\" -> 0.000000000000   ,  \"Reoff\" -> -17138775.510204076800   ,  \"Imoff\" -> 0.000000000000   ,  \"στ1\" -> 0.002172719957   ,  \"στS\" -> 0.000093763545   ,  \"στN\" -> 0.000355038458   ,  \"τ11 \" -> 0.000000000000   ,  \"τ12\" -> 0.000000000000   ,  \"τ22\" -> 0.000000000000   ,  \"τN1\" -> 0.000000000000   ,  \"τN2\" -> 0.000000000000   ,  \"σηlogτ1 \" -> 0.000000000000   ,  \"σηlogτS\" -> 0.000000000000   ,  \"σηlogτN\" -> 0.000000000000   ,  \"σlogτ1\" -> 0.000000000000   ,  \"σlogτS\" -> 0.000000000000   ,  \"σlogτN\" -> 0.000000000000   ,  \"σητ1\" -> 0.000000000000   ,  \"σητS \" -> 0.000000000000   ,  \"σητN\" -> 0.000000000000    |>   , \r\"IDS0409_220525_RAW_cal__sam_\" ->   <|    \"ζ\" -> 0.056561047780   ,  \"τ1\" -> 0.014299678758   ,  \"τS\" -> 0.013769239985   ,  \"τN\" -> 0.003071380883   ,  \"τC\" -> 0.001651608796   ,  \"κ0\" -> 0.000000001520   ,  \"mm1\" -> 0.000079784788   ,  \"mm2\" -> 0.009566648569   ,  \"mm3\" -> 0.024097998227   ,  \"T\" -> 0.300000000000   ,  \"B\" -> 0.000000000000   ,  \"θ\" -> 0.000000000000   ,  \"Reoff\" -> -9836734.693877555430   ,  \"Imoff\" -> 0.000000000000   ,  \"στ1\" -> 0.019869000982   ,  \"στS\" -> 0.002333902836   ,  \"στN\" -> 0.003131938876   ,  \"τ11 \" -> 0.000000000000   ,  \"τ12\" -> 0.000000000000   ,  \"τ22\" -> 0.000000000000   ,  \"τN1\" -> 0.000000000000   ,  \"τN2\" -> 0.000000000000   ,  \"σηlogτ1 \" -> 0.000000000000   ,  \"σηlogτS\" -> 0.000000000000   ,  \"σηlogτN\" -> 0.000000000000   ,  \"σlogτ1\" -> 0.000000000000   ,  \"σlogτS\" -> 0.000000000000   ,  \"σlogτN\" -> 0.000000000000   ,  \"σητ1\" -> 0.000000000000   ,  \"σητS \" -> 0.000000000000   ,  \"σητN\" -> 0.000000000000    |>   , \r\"IDS0410_220525_RAW_cal__ref_\" ->   <|    \"ζ\" -> 0.219464822230   ,  \"τ1\" -> 0.031337357476   ,  \"τS\" -> 0.015000716363   ,  \"τN\" -> 0.006678392144   ,  \"τC\" -> 0.001899192874   ,  \"κ0\" -> 0.000000000590   ,  \"mm1\" -> 0.000314430704   ,  \"mm2\" -> 0.013625332075   ,  \"mm3\" -> 0.045733697773   ,  \"T\" -> 0.170000000000   ,  \"B\" -> 0.000000000000   ,  \"θ\" -> 0.000000000000   ,  \"Reoff\" -> -36285714.285714283600   ,  \"Imoff\" -> 0.000000000000   ,  \"στ1\" -> 0.008766031660   ,  \"στS\" -> 0.001214804635   ,  \"στN\" -> 0.000507557698   ,  \"τ11 \" -> 0.000000000000   ,  \"τ12\" -> 0.000000000000   ,  \"τ22\" -> 0.000000000000   ,  \"τN1\" -> 0.000000000000   ,  \"τN2\" -> 0.000000000000   ,  \"σηlogτ1 \" -> 0.000000000000   ,  \"σηlogτS\" -> 0.000000000000   ,  \"σηlogτN\" -> 0.000000000000   ,  \"σlogτ1\" -> 0.000000000000   ,  \"σlogτS\" -> 0.000000000000   ,  \"σlogτN\" -> 0.000000000000   ,  \"σητ1\" -> 0.000000000000   ,  \"σητS \" -> 0.000000000000   ,  \"σητN\" -> 0.000000000000    |>   , \r\"IDS0410_220525_RAW_cal__sam_\" ->   <|    \"ζ\" -> 0.124885425459   ,  \"τ1\" -> 0.026966294273   ,  \"τS\" -> 0.017799663974   ,  \"τN\" -> 0.005835531331   ,  \"τC\" -> 0.001338388753   ,  \"κ0\" -> 0.000000000710   ,  \"mm1\" -> 0.000140185240   ,  \"mm2\" -> 0.014066781222   ,  \"mm3\" -> 0.040684603290   ,  \"T\" -> 0.170000000000   ,  \"B\" -> 0.000000000000   ,  \"θ\" -> 0.000000000000   ,  \"Reoff\" -> -36285714.285714283600   ,  \"Imoff\" -> 0.000000000000   ,  \"στ1\" -> 0.125291630718   ,  \"στS\" -> 0.008513087182   ,  \"στN\" -> 0.016544280517   ,  \"τ11 \" -> 0.000000000000   ,  \"τ12\" -> 0.000000000000   ,  \"τ22\" -> 0.000000000000   ,  \"τN1\" -> 0.000000000000   ,  \"τN2\" -> 0.000000000000   ,  \"σηlogτ1 \" -> 0.000000000000   ,  \"σηlogτS\" -> 0.000000000000   ,  \"σηlogτN\" -> 0.000000000000   ,  \"σlogτ1\" -> 0.000000000000   ,  \"σlogτS\" -> 0.000000000000   ,  \"σlogτN\" -> 0.000000000000   ,  \"σητ1\" -> 0.000000000000   ,  \"σητS \" -> 0.000000000000   ,  \"σητN\" -> 0.000000000000    |>   , \r\"IDS0411_220525_RAW_cal__ref_\" ->   <|    \"ζ\" -> 0.246063307500   ,  \"τ1\" -> 0.040789582366   ,  \"τS\" -> 0.016746728194   ,  \"τN\" -> 0.008396680213   ,  \"τC\" -> 0.002075116481   ,  \"κ0\" -> 0.000000000510   ,  \"mm1\" -> 0.000378838091   ,  \"mm2\" -> 0.015895872639   ,  \"mm3\" -> 0.057920266758   ,  \"T\" -> 0.150000000000   ,  \"B\" -> 0.000000000000   ,  \"θ\" -> 0.000000000000   ,  \"Reoff\" -> -36285714.285714283600   ,  \"Imoff\" -> 0.000000000000   ,  \"στ1\" -> 0.014361572724   ,  \"στS\" -> 0.001491857642   ,  \"στN\" -> 0.002913772081   ,  \"τ11 \" -> 0.000000000000   ,  \"τ12\" -> 0.000000000000   ,  \"τ22\" -> 0.000000000000   ,  \"τN1\" -> 0.000000000000   ,  \"τN2\" -> 0.000000000000   ,  \"σηlogτ1 \" -> 0.000000000000   ,  \"σηlogτS\" -> 0.000000000000   ,  \"σηlogτN\" -> 0.000000000000   ,  \"σlogτ1\" -> 0.000000000000   ,  \"σlogτS\" -> 0.000000000000   ,  \"σlogτN\" -> 0.000000000000   ,  \"σητ1\" -> 0.000000000000   ,  \"σητS \" -> 0.000000000000   ,  \"σητN\" -> 0.000000000000    |>   , \r\"IDS0411_220525_RAW_cal__sam_\" ->   <|    \"ζ\" -> 0.135609092663   ,  \"τ1\" -> 0.033619209304   ,  \"τS\" -> 0.020242350677   ,  \"τN\" -> 0.009065316224   ,  \"τC\" -> 0.001338388753   ,  \"κ0\" -> 0.000000000610   ,  \"mm1\" -> 0.000151964902   ,  \"mm2\" -> 0.015437467353   ,  \"mm3\" -> 0.052650218819   ,  \"T\" -> 0.150000000000   ,  \"B\" -> 0.000000000000   ,  \"θ\" -> 0.000000000000   ,  \"Reoff\" -> -36285714.285714283600   ,  \"Imoff\" -> 0.000000000000   ,  \"στ1\" -> 0.012006153279   ,  \"στS\" -> 0.002506054906   ,  \"στN\" -> 0.002275285607   ,  \"τ11 \" -> 0.000000000000   ,  \"τ12\" -> 0.000000000000   ,  \"τ22\" -> 0.000000000000   ,  \"τN1\" -> 0.000000000000   ,  \"τN2\" -> 0.000000000000   ,  \"σηlogτ1 \" -> 0.000000000000   ,  \"σηlogτS\" -> 0.000000000000   ,  \"σηlogτN\" -> 0.000000000000   ,  \"σlogτ1\" -> 0.000000000000   ,  \"σlogτS\" -> 0.000000000000   ,  \"σlogτN\" -> 0.000000000000   ,  \"σητ1\" -> 0.000000000000   ,  \"σητS \" -> 0.000000000000   ,  \"σητN\" -> 0.000000000000    |>   , \r\"IDS0412_220525_RAW_cal__ref_\" ->   <|    \"ζ\" -> 0.277356261420   ,  \"τ1\" -> 0.054222210065   ,  \"τS\" -> 0.019549661431   ,  \"τN\" -> 0.015941590375   ,  \"τC\" -> 0.002328566298   ,  \"κ0\" -> 0.000000000395   ,  \"mm1\" -> 0.000470356932   ,  \"mm2\" -> 0.017304710415   ,  \"mm3\" -> 0.084110681736   ,  \"T\" -> 0.120000000000   ,  \"B\" -> 0.000000000000   ,  \"θ\" -> 0.000000000000   ,  \"Reoff\" -> -36285714.285714283600   ,  \"Imoff\" -> 0.000000000000   ,  \"στ1\" -> 0.003181743448   ,  \"στS\" -> 0.002733063927   ,  \"στN\" -> 0.005931070528   ,  \"τ11 \" -> 0.000000000000   ,  \"τ12\" -> 0.000000000000   ,  \"τ22\" -> 0.000000000000   ,  \"τN1\" -> 0.000000000000   ,  \"τN2\" -> 0.000000000000   ,  \"σηlogτ1 \" -> 0.000000000000   ,  \"σηlogτS\" -> 0.000000000000   ,  \"σηlogτN\" -> 0.000000000000   ,  \"σlogτ1\" -> 0.000000000000   ,  \"σlogτS\" -> 0.000000000000   ,  \"σlogτN\" -> 0.000000000000   ,  \"σητ1\" -> 0.000000000000   ,  \"σητS \" -> 0.000000000000   ,  \"σητN\" -> 0.000000000000    |>   , \r\"IDS0412_220525_RAW_cal__sam_\" ->   <|    \"ζ\" -> 0.141872667412   ,  \"τ1\" -> 0.045522682755   ,  \"τS\" -> 0.024683404671   ,  \"τN\" -> 0.014187266741   ,  \"τC\" -> 0.001029575567   ,  \"κ0\" -> 0.000000000485   ,  \"mm1\" -> 0.000123931838   ,  \"mm2\" -> 0.018251391889   ,  \"mm3\" -> 0.072562291843   ,  \"T\" -> 0.120000000000   ,  \"B\" -> 0.000000000000   ,  \"θ\" -> 0.000000000000   ,  \"Reoff\" -> -36285714.285714283600   ,  \"Imoff\" -> 0.000000000000   ,  \"στ1\" -> 0.019575103663   ,  \"στS\" -> 0.006297786999   ,  \"στN\" -> 0.007663344539   ,  \"τ11 \" -> 0.000000000000   ,  \"τ12\" -> 0.000000000000   ,  \"τ22\" -> 0.000000000000   ,  \"τN1\" -> 0.000000000000   ,  \"τN2\" -> 0.000000000000   ,  \"σηlogτ1 \" -> 0.000000000000   ,  \"σηlogτS\" -> 0.000000000000   ,  \"σηlogτN\" -> 0.000000000000   ,  \"σlogτ1\" -> 0.000000000000   ,  \"σlogτS\" -> 0.000000000000   ,  \"σlogτN\" -> 0.000000000000   ,  \"σητ1\" -> 0.000000000000   ,  \"σητS \" -> 0.000000000000   ,  \"σητN\" -> 0.000000000000    |>   , \r\"IDS0413_220525_RAW_cal__ref_\" ->   <|    \"ζ\" -> 0.078611813010   ,  \"τ1\" -> 0.009498211202   ,  \"τS\" -> 0.010412643153   ,  \"τN\" -> 0.002291796830   ,  \"τC\" -> 0.001202807939   ,  \"κ0\" -> 0.000000001750   ,  \"mm1\" -> 0.000079680552   ,  \"mm2\" -> 0.006634465733   ,  \"mm3\" -> 0.017690031900   ,  \"T\" -> 0.360000000000   ,  \"B\" -> 0.000000000000   ,  \"θ\" -> 0.000000000000   ,  \"Reoff\" -> -10542857.142857149200   ,  \"Imoff\" -> 0.000000000000   ,  \"στ1\" -> 0.000920556157   ,  \"στS\" -> 0.001775574992   ,  \"στN\" -> 0.000302317441   ,  \"τ11 \" -> 0.000000000000   ,  \"τ12\" -> 0.000000000000   ,  \"τ22\" -> 0.000000000000   ,  \"τN1\" -> 0.000000000000   ,  \"τN2\" -> 0.000000000000   ,  \"σηlogτ1 \" -> 0.000000000000   ,  \"σηlogτS\" -> 0.000000000000   ,  \"σηlogτN\" -> 0.000000000000   ,  \"σlogτ1\" -> 0.000000000000   ,  \"σlogτS\" -> 0.000000000000 
